vi "Create Frame.vi"() -> (0 "Color":u32(colorbox), 1 "Max Available Position":refnum<class "Vector2.lvclass">, 2 "Min Available Position":refnum<class "Vector2.lvclass">, 3 "Simulation Objects":refnum<class "SimulationObject.lvclass">[](array[class]))   [LabVIEW 2022 SP3]
uses:
  Engine/Objects/SimulationObject/SimulationObject.lvclass
  Engine/Math/Vector2/Vector2.lvclass
  Engine/Objects/SimulationObject/SimulationObject.lvclass/SimulationObject.ctl
  Engine/Objects/Components/PhysicsComponent/PhysicsComponent.lvclass/PhysicsComponent.ctl
  Engine/Objects/Shapes/RectangleShape/RectangleShape.lvclass
  D:/Programowanie/Studia/Labview/CollisionSimulator/Project/Engine/Objects/Shapes/Shapeable/Shapeable.lvclass
  Engine/Objects/Components/PhysicsComponent/PhysicsComponent.lvclass
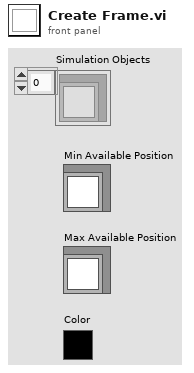
[diagram p1: front panel]
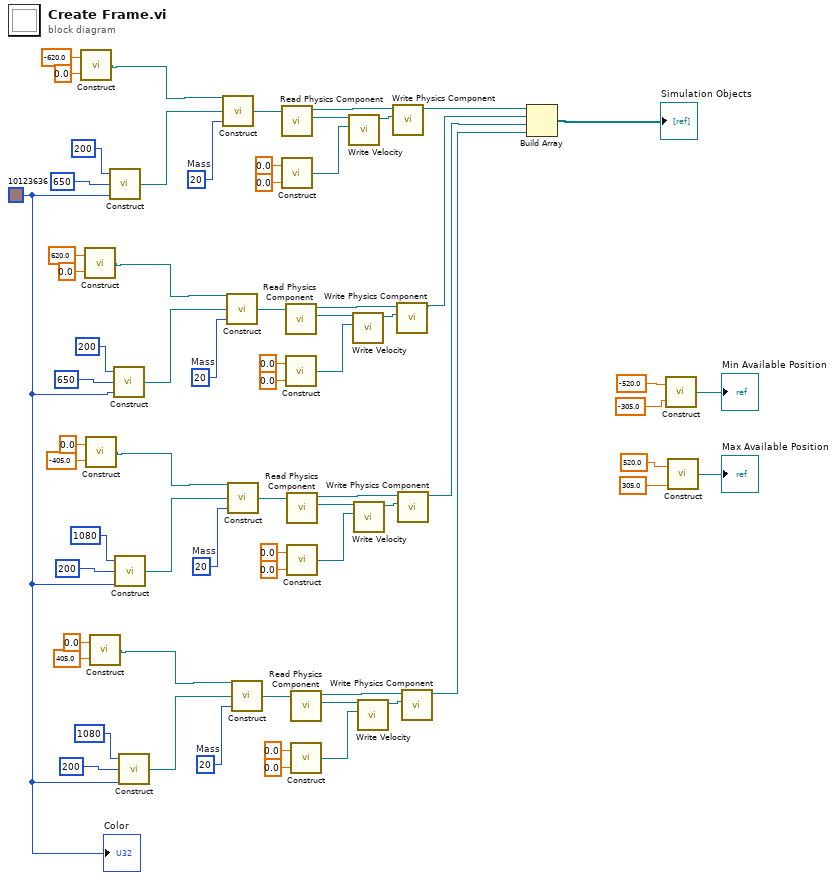
[diagram p0: block diagram]
diagram:
  w19 = 20  # Mass
  w33 = 20  # Mass
  w47 = 20  # Mass
  w7 = u32 10123636 ("Color")
  w61 = 20  # Mass
  n1 = call "Construct.vi"("y"=sgl 0.0, "x"=sgl -620.0) -> ("Vec2 out"=w60:refnum<class "Vector2.lvclass">)
  n2 = call "Construct.vi"("y"=sgl 0.0, "x"=sgl 620.0) -> ("Vec2 out"=w46:refnum<class "Vector2.lvclass">)
  n3 = call "Construct.vi"("y"=sgl -405.0, "x"=sgl 0.0) -> ("Vec2 out"=w32:refnum<class "Vector2.lvclass">)
  n4 = call "Construct.vi"("y"=sgl 405.0, "x"=sgl 0.0) -> ("Vec2 out"=w18:refnum<class "Vector2.lvclass">)
  n5 = call "Construct.vi"("Color"=w7, "Height"=i16 650, "Width"=i16 200) -> ("RectangleShape out"=w57:refnum<class "RectangleShape.lvclass">)
  n6 = call "Construct.vi"("Color"=w7, "Height"=i16 650, "Width"=i16 200) -> ("RectangleShape out"=w43:refnum<class "RectangleShape.lvclass">)
  n7 = call "Construct.vi"("Color"=w7, "Height"=i16 200, "Width"=i16 1080) -> ("RectangleShape out"=w29:refnum<class "RectangleShape.lvclass">)
  n8 = call "Construct.vi"("Color"=w7, "Height"=i16 200, "Width"=i16 1080) -> ("RectangleShape out"=w15:refnum<class "RectangleShape.lvclass">)
  n9 = call "Construct.vi"("Mass"=w61, "Shape in"=w57, "Local Position in"=w60) -> ("Simulation Object out"=w62:refnum<class "SimulationObject.lvclass">)
  n10 = call "Construct.vi"("Mass"=w47, "Shape in"=w43, "Local Position in"=w46) -> ("Simulation Object out"=w48:refnum<class "SimulationObject.lvclass">)
  n11 = call "Construct.vi"("Mass"=w33, "Shape in"=w29, "Local Position in"=w32) -> ("Simulation Object out"=w34:refnum<class "SimulationObject.lvclass">)
  n12 = call "Construct.vi"("Mass"=w19, "Shape in"=w15, "Local Position in"=w18) -> ("Simulation Object out"=w20:refnum<class "SimulationObject.lvclass">)
  n13 = call "Read Physics Component.vi"("SimulationObject in"=w62) -> ("Physics Component out"=w65:refnum<class "PhysicsComponent.lvclass">, "SimulationObject out"=w63:refnum<class "SimulationObject.lvclass">)  [unwired: 8 in, 1 out]
  n14 = call "Construct.vi"("y"=sgl 0.0, "x"=sgl 0.0) -> ("Vec2 out"=w66:refnum<class "Vector2.lvclass">)
  n15 = call "Read Physics Component.vi"("SimulationObject in"=w48) -> ("Physics Component out"=w51:refnum<class "PhysicsComponent.lvclass">, "SimulationObject out"=w49:refnum<class "SimulationObject.lvclass">)  [unwired: 8 in, 1 out]
  n16 = call "Construct.vi"("y"=sgl 0.0, "x"=sgl 0.0) -> ("Vec2 out"=w52:refnum<class "Vector2.lvclass">)
  n17 = call "Read Physics Component.vi"("SimulationObject in"=w34) -> ("Physics Component out"=w37:refnum<class "PhysicsComponent.lvclass">, "SimulationObject out"=w35:refnum<class "SimulationObject.lvclass">)  [unwired: 8 in, 1 out]
  n18 = call "Construct.vi"("y"=sgl 0.0, "x"=sgl 0.0) -> ("Vec2 out"=w38:refnum<class "Vector2.lvclass">)
  n19 = call "Read Physics Component.vi"("SimulationObject in"=w20) -> ("Physics Component out"=w23:refnum<class "PhysicsComponent.lvclass">, "SimulationObject out"=w21:refnum<class "SimulationObject.lvclass">)  [unwired: 8 in, 1 out]
  n20 = call "Construct.vi"("y"=sgl 0.0, "x"=sgl 0.0) -> ("Vec2 out"=w24:refnum<class "Vector2.lvclass">)
  n21 = call "Write Velocity.vi"("Velocity in"=w66, "PhysicsComponent in"=w65) -> ("PhysicsComponent out"=w64:refnum<class "PhysicsComponent.lvclass">)  [unwired: 8 in, 1 out]
  n22 = call "Write Velocity.vi"("Velocity in"=w52, "PhysicsComponent in"=w51) -> ("PhysicsComponent out"=w50:refnum<class "PhysicsComponent.lvclass">)  [unwired: 8 in, 1 out]
  n23 = call "Write Velocity.vi"("Velocity in"=w38, "PhysicsComponent in"=w37) -> ("PhysicsComponent out"=w36:refnum<class "PhysicsComponent.lvclass">)  [unwired: 8 in, 1 out]
  n24 = call "Write Velocity.vi"("Velocity in"=w24, "PhysicsComponent in"=w23) -> ("PhysicsComponent out"=w22:refnum<class "PhysicsComponent.lvclass">)  [unwired: 8 in, 1 out]
  n25 = call "Write Physics Component.vi"("PhysicsComponent.lvclass"=w64, "SimulationObject in"=w63) -> ("SimulationObject out"=w12:refnum<class "SimulationObject.lvclass">)  [unwired: 8 in, 1 out]
  n26 = call "Write Physics Component.vi"("PhysicsComponent.lvclass"=w50, "SimulationObject in"=w49) -> ("SimulationObject out"=w11:refnum<class "SimulationObject.lvclass">)  [unwired: 8 in, 1 out]
  n27 = call "Write Physics Component.vi"("PhysicsComponent.lvclass"=w36, "SimulationObject in"=w35) -> ("SimulationObject out"=w10:refnum<class "SimulationObject.lvclass">)  [unwired: 8 in, 1 out]
  n28 = call "Write Physics Component.vi"("PhysicsComponent.lvclass"=w22, "SimulationObject in"=w21) -> ("SimulationObject out"=w9:refnum<class "SimulationObject.lvclass">)  [unwired: 8 in, 1 out]
  n29 = Build Array(w12, w11, w10, w9) -> (→"Simulation Objects":refnum<class "SimulationObject.lvclass">[])
  n30 = call "Construct.vi"("y"=sgl -305.0 ("x"), "x"=sgl -520.0) -> ("Vec2 out"=→"Min Available Position":refnum<class "Vector2.lvclass">)
  n31 = call "Construct.vi"("y"=sgl 305.0 ("x"), "x"=sgl 520.0) -> ("Vec2 out"=→"Max Available Position":refnum<class "Vector2.lvclass">)
  "Color" <- w7
